vi "ElevLimit.vi"(11 "PowerIn":dbl) -> (2 "BotLimit":bool, 3 "PowerOut":dbl, 5 "UpLimit":bool)   [LabVIEW 2018]
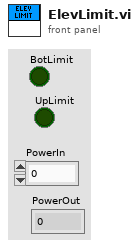
[diagram p1: front panel]
types:
  T1 = typedef "WPI_SwitchDevRef.ctl" = cluster{"DevStatus":errorcluster, "DIO Channel":T2, "CntIndex":T3, "Normally Closed":bool}
  T2 = typedef "FPGA_DIOChannel.ctl" = enum8{"DIO 0", "DIO 1", "DIO 2", "DIO 3", "DIO 4", "DIO 5", "DIO 6", "DIO 7", "DIO 8", "DIO 9", "DIO MXP 0", "DIO MXP 1", "DIO MXP 2", "DIO MXP 3", "DIO MXP 4", "DIO MXP 5", "DIO MXP 6", "DIO MXP 7", "DIO MXP 8", "DIO MXP 9", "DIO MXP 10", "DIO MXP 11", "DIO MXP 12", "DIO MXP 13", "DIO MXP 14", "DIO MXP 15", "SPI Port CS1", "SPI Port CS2", "SPI Port CS3", "SPI Port MISO", "SPI Port MOSI", "Invalid"}
  T3 = typedef "FPGA_CounterCtrSystemIndex.ctl" = enum8{"Ctr 0", "Ctr 1", "Ctr 2", "Ctr 3", "Ctr 4", "Ctr 5", "Ctr 6", "Ctr 7", "Invalid"}
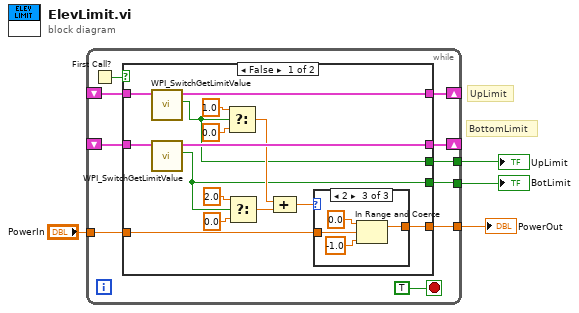
[diagram p0: block diagram]
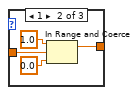
[diagram p3: hidden frame]
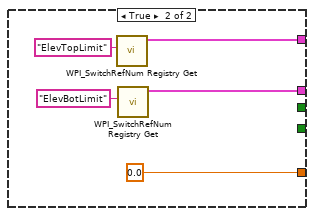
[diagram p4: hidden frame]
diagram:
  # "BottomLimit"
  # "UpLimit"
  n1 = while {
    shift-right: [w11] -> _
    shift-left: _ -> [w9]
    shift-right: [w12] -> _
    shift-left: _ -> [w10]
    tunnel: "PowerIn" -> [w8]
    tunnel: [w7] -> w1
    tunnel: [w6] -> w4
    tunnel: [w5] -> w3
    stop <- TRUE stop-if-true
    n2 = First Call?() -> (First Call?: T/F=w13:bool)
    n3 = case shown="False" w13 {
      tunnel: [w26 w41] -> w12
      tunnel: [w28 w40] -> w11
      tunnel: w10 -> [w27 _]
      tunnel: w9 -> [w29 _]
      tunnel: w8 -> [w18 _]
      tunnel: [w17 0.0 ("upper limit")] -> w7
      tunnel: [w16 _] -> w6
      tunnel: [w15 _] -> w5
      frame False {
        n4 = call <vilib>:"WPI_SwitchGetLimitValue.vi"("SwitchDevRef"=w29) -> ("Switch Pressed"=w15:bool, "SwitchDevRef"=w28:T1)  [unwired: 8 in, 1 out]
        n5 = call <vilib>:"WPI_SwitchGetLimitValue.vi"("SwitchDevRef"=w27) -> ("Switch Pressed"=w16:bool, "SwitchDevRef"=w26:T1)  [unwired: 8 in, 1 out]
        n6 = Select(t=1.0, s=w15, f=0.0) -> (s? t:f=w22:dbl)
        n7 = Select(t=2.0, s=w16, f=0.0) -> (s? t:f=w19:dbl)
        n8 = Compound Arithmetic op=ADD(w22, w19) -> (w25:dbl)
        n9 = case shown="2" w25 {
          tunnel: w18 -> [w30 w34 w38]
          tunnel: [w30 w33 w35] -> w17
          frame 0, Default {
          }
          frame 1 {
            n10 = In Range and Coerce(upper limit=1.0, x=w34, lower limit=0.0) -> (coerced(x)=w33:dbl)  [unwired: 1 out]
          }
          frame 2 {
            n11 = In Range and Coerce(upper limit=0.0, x=w38, lower limit=-1.0) -> (coerced(x)=w35:dbl)  [unwired: 1 out]
          }
        }
      }
      frame True {
        n12 = call <vilib>:"WPI_SwitchRefNum Registry Get.vi"("refnum name"="ElevTopLimit") -> ("SwitchDevRef"=w40:T1)  [unwired: 9 in, 1 out]
        n13 = call <vilib>:"WPI_SwitchRefNum Registry Get.vi"("refnum name"="ElevBotLimit") -> ("SwitchDevRef"=w41:T1)  [unwired: 9 in, 1 out]
      }
    }
  }
  "BotLimit" <- w4
  "UpLimit" <- w3
  "PowerOut" <- w1
